vi "pack_map_len.vi"(3 "error in":errorcluster, 4 "n":u32, 5 "p":u64) -> (0 "error out":errorcluster, 2 "p out":u64)   [LabVIEW 2019, in "msgpack.lvlib"]
doc: "Packs a header into the buffer indicating the start of an associative array (\"map\").\n\nFollowing this call you are then required to write 2N objects, corresponding to keys interleaved with values.\n\nUse the pack_cluster VI for a convenience wrapper around this function."
uses:
  msgpack.lvlib
  msgpackalt.dll
panel:
  # "msgpack"
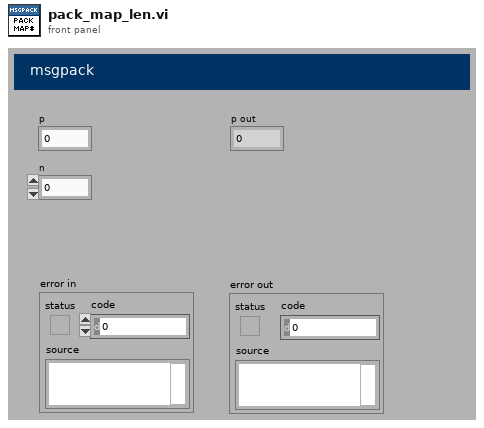
[diagram p1: front panel]
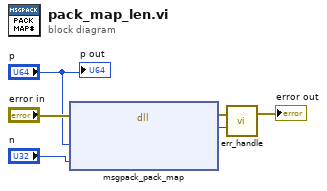
[diagram p0: block diagram]
diagram:
  n1 = dll-call lib="C:/Users/Patrick/Documents/GitHub/Instrument-Framework/lvsrc/SMOs/JSON-RPC-2019/lv-venv/lv.lib/vi.lib/addons/msgpack/msgpackalt.dll" fn="msgpack_pack_map"(error in="error in", "p"="p", "n"="n") -> (error out=w3:errorcluster, "return type"=w4:i32)  [unwired: 4 in, 1 out]
  n2 = call "err_handle.vi"("retval"=w4, "error in"=w3) -> ("error out"=→"error out":errorcluster)  [unwired: 1 in]
  "p out" <- "p"
